vi "Read AppOutput.vi"(8 "error in (no error)":errorcluster, 11 "VisualizeAppBase_class in":refnum<class "VisualizeAppBase_class.lvclass">) -> (0 "error out":errorcluster, 2 "AppOutput":variant, 3 "VisualizeAppBase_class out":refnum<class "VisualizeAppBase_class.lvclass">)   [LabVIEW 2014]
uses:
  VisualizeAppBase_class.lvclass
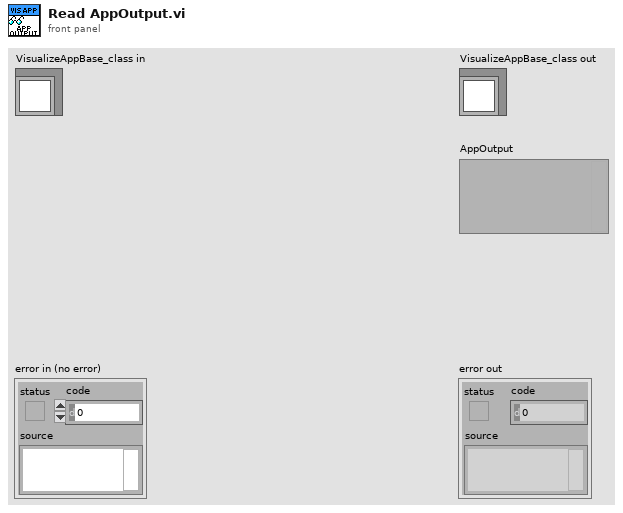
[diagram p1: front panel]
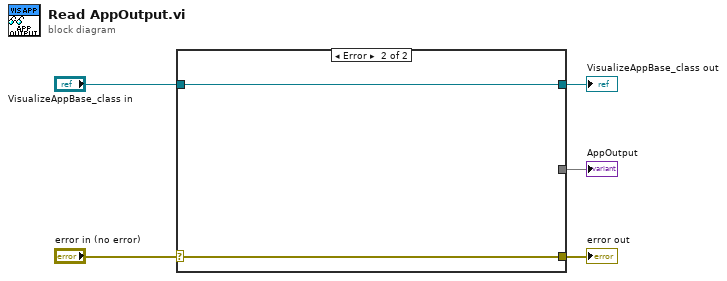
[diagram p0: block diagram]
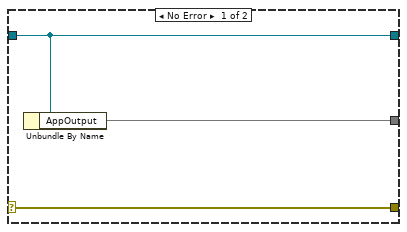
[diagram p2: hidden frame]
diagram:
  n1 = case shown="Error" "error in (no error)" {
    selector: "error in (no error)" -> [w8 w9]
    tunnel: [w8 w9] -> w4
    tunnel: [w7 w10] -> w2
    tunnel: "VisualizeAppBase_class in" -> [w7 w10]
    tunnel: [w6 _] -> w1
    frame No Error {
      n2 = Unbundle By Name(w7) -> ("AppOutput"=w6)
    }
    frame Error {
    }
  }
  "error out" <- w4
  "VisualizeAppBase_class out" <- w2
  "AppOutput" <- w1
